vi "Open Queue.vi"(8 "error in (no error)":errorcluster, 11 "DbMeasurement in":refnum<class "DbMeasurement.lvclass">) -> (0 "error out":errorcluster, 3 "DbMeasurement out":refnum<class "DbMeasurement.lvclass">)   [LabVIEW 2013, in "DbMeasurement.lvclass"]
doc: "This private method obtains a queue for the variant data type used for database values."
uses:
  DbMeasurement.lvclass
  DbMeasurement.lvclass/DbMeasurement.ctl
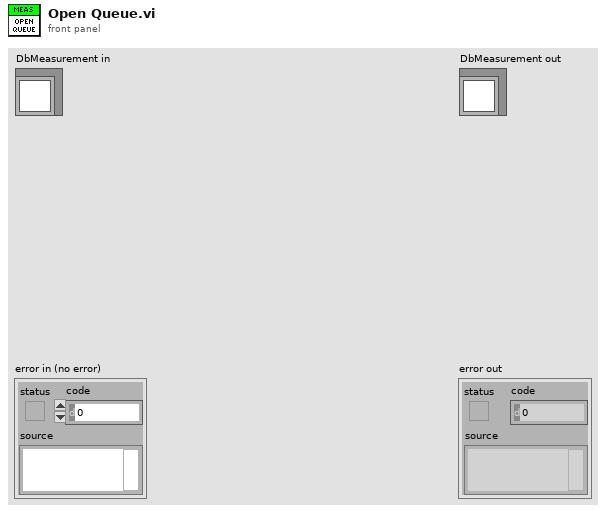
[diagram p1: front panel]
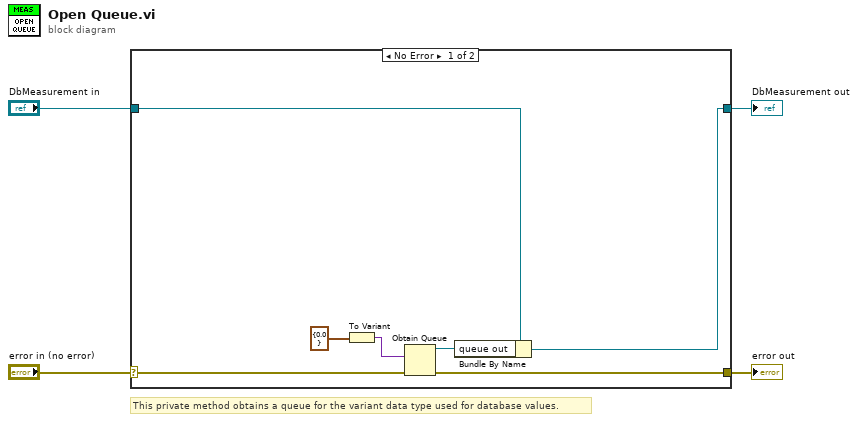
[diagram p0: block diagram]
diagram:
  # "This private method obtains a queue for the variant data type used for database values."
  n1 = case shown="No Error" "error in (no error)" {
    selector: "error in (no error)" -> [w11 w13]
    tunnel: [w10 w13] -> w3
    tunnel: [w5 w12] -> w1
    tunnel: "DbMeasurement in" -> [w9 w12]
    frame No Error {
      n2 = To Variant(anything=cluster{dbl} {0.0}) -> (Variant=w7:variant)
      n3 = Obtain Queue(element data type=w7, error in (no error)=w11) -> (queue out=w6:refnum<queue>, error out=w10:errorcluster)  [unwired: 3 in, 1 out]
      n4 = Bundle By Name(cluster=w9, "queue out"=w6) -> (w5:refnum<class "DbMeasurement.lvclass">)
    }
    frame Error {
    }
  }
  "error out" <- w3
  "DbMeasurement out" <- w1
